vi "CHP Measure.vi"(0 "Instrument Handle In":refnum<k21>, 5 "Harm Timeout (s)":dbl=10.0 format="%.3f", 11 "error in (no error)":errorcluster) -> (4 "Instrument Handle Out":refnum<k21>, 6 "CHP Results":T1 {"Total Carrier Power (dBm)" format="%.2f"; "Peak Amplitude (dBm/Hz)" format="%.2f"}, 15 "error out":errorcluster)   [LabVIEW 2016, in "RFmxSpecAn.lvlib"]
uses:
  RFmxSpecAn.lvlib
  <vilib>/RFmx/SpecAn/mx/RFmxSpecAn.llb/RFmxSpecAn Select Measurement (Multiple).vi
  <vilib>/RFmx/SpecAn/mx/RFmxSpecAn.llb/RFmxSpecAn CHP Fetch Total Carrier Power.vi
  <vilib>/RFmx/SpecAn/mx/RFmxSpecAn.llb/RFmxSpecAn Spectrum Fetch Measurement.vi
  <vilib>/RFmx/SpecAn/mx/RFmxSpecAn.llb/RFmxSpecAn CHP Fetch Spectrum.vi
  Typedefs/CHP Results.ctl
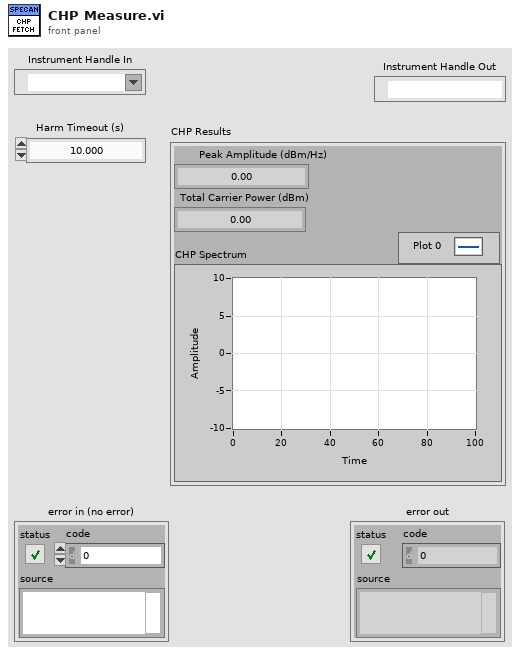
[diagram p1: front panel]
types:
  T1 = typedef "RFmxSpecAn.lvlib/CHP Results.ctl" = cluster{"Peak Amplitude (dBm/Hz)":dbl, "Total Carrier Power (dBm)":dbl, "CHP Spectrum":cluster{"x0":dbl, "dx":dbl, "y":sgl[]}}
  T2 = enum16{"ACP", "CCDF", "CHP", "FCnt", "Harmonics", "OBW", "SEM", "Spectrum", "Spur", "TXP", "AMPM", "DPD", "IQ", "IM", "NF", "PhaseNoise"}[]
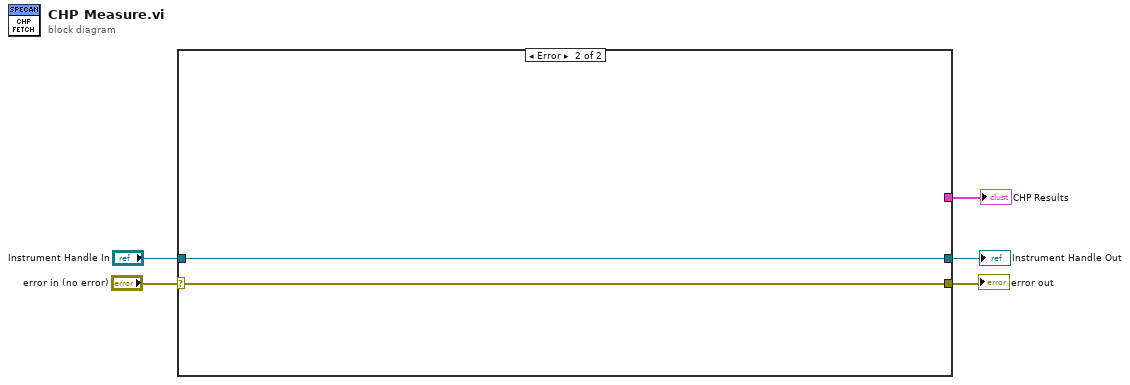
[diagram p0: block diagram]
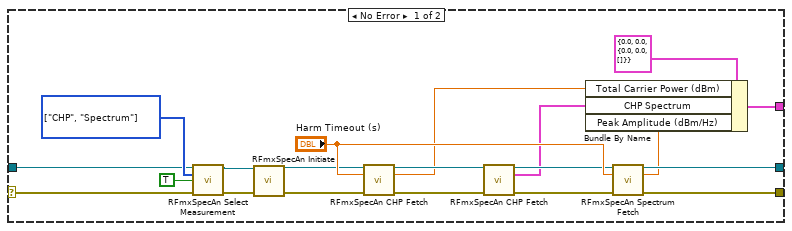
[diagram p2: hidden frame]
diagram:
  n1 = case shown="Error" "error in (no error)" {
    selector: "error in (no error)" -> [w6 w26]
    tunnel: "Instrument Handle In" -> [w18 w27]
    tunnel: [w17 w27] -> w4
    tunnel: [w16 w26] -> w3
    tunnel: [w7 _] -> w2
    frame No Error {
      w22 = T2 [enum."CHP", enum."Spectrum"] items=["ACP", "CCDF", "CHP", "FCnt", "Harmonics", "OBW", "SEM", "Spectrum", "Spur", "TXP", "AMPM", "DPD", "IQ", "IM", "NF", "PhaseNoise"]
      n2 = call-poly <vilib>:"RFmxSpecAn Select Measurement.vi"("Instrument Handle In"=w18, "Measurements"=w22, "Enable All Traces"=TRUE, "error in (no error)"=w6) -> ("Instrument Handle Out"=w19:refnum<k21>, "error out"=w20:errorcluster)  [unwired: 10 in]
      n3 = call <vilib>:"RFmxSpecAn Initiate.vi"("Instrument Handle In"=w19, "error in (no error)"=w20) -> ("Instrument Handle Out"=w23:refnum<k21>, "error out"=w24:errorcluster)  [unwired: 11 in, 1 out]
      n4 = call-poly <vilib>:"RFmxSpecAn CHP Fetch.vi"("Instrument Handle In"=w23, "Timeout (s)"="Harm Timeout (s)", "error in (no error)"=w24) -> ("Instrument Handle Out"=w15:refnum<k21>, "Total Carrier Power (dBm)"=w10:dbl, "error out"=w14:errorcluster)  [unwired: 10 in]
      n5 = call-poly <vilib>:"RFmxSpecAn CHP Fetch.vi"("Instrument Handle In"=w15, "error in (no error)"=w14) -> ("Instrument Handle Out"=w12:refnum<k21>, "Spectrum (dBm)"=w9:cluster{"x0":dbl, "dx":dbl, "y":sgl[]}, "error out"=w13:errorcluster)  [unwired: 11 in]
      n6 = call-poly <vilib>:"RFmxSpecAn Spectrum Fetch.vi"("Instrument Handle In"=w12, "Timeout (s)"="Harm Timeout (s)", "error in (no error)"=w13) -> ("Instrument Handle Out"=w17:refnum<k21>, "Peak Amplitude"=w8:dbl, "error out"=w16:errorcluster)  [unwired: 8 in, 2 out]
      n7 = Bundle By Name(cluster=T1 {"Peak Amplitude (dBm/Hz)"=0.0, "Total Carrier Power (dBm)"=0.0, "CHP Spectrum"={"x0"=0.0, "dx"=0.0, "y"=[]}} ("CHP Results"), "Total Carrier Power (dBm)"=w10, "CHP Spectrum"=w9, "Peak Amplitude (dBm/Hz)"=w8) -> (w7:T1)
    }
    frame Error {
    }
  }
  "Instrument Handle Out" <- w4
  "error out" <- w3
  "CHP Results" <- w2
